vi "MT_generate_signal5.vi"(7 "Direction":bool, 8 "error in (no error)":errorcluster, 9 "# cycles":dbl, 10 "frequency":dbl, 11 "amplitude":dbl) -> (0 "error out":errorcluster, 2 "signals out":dbl[][](array[numeric]), 3 "# samples":dbl)   [LabVIEW 2019]
uses:
  <vilib>/Analysis/NI_AALBase.lvlib
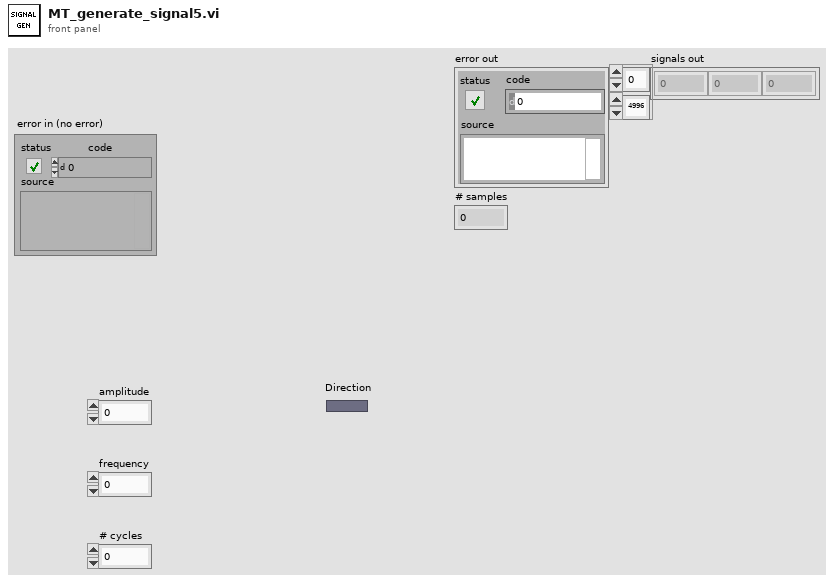
[diagram p1: front panel]
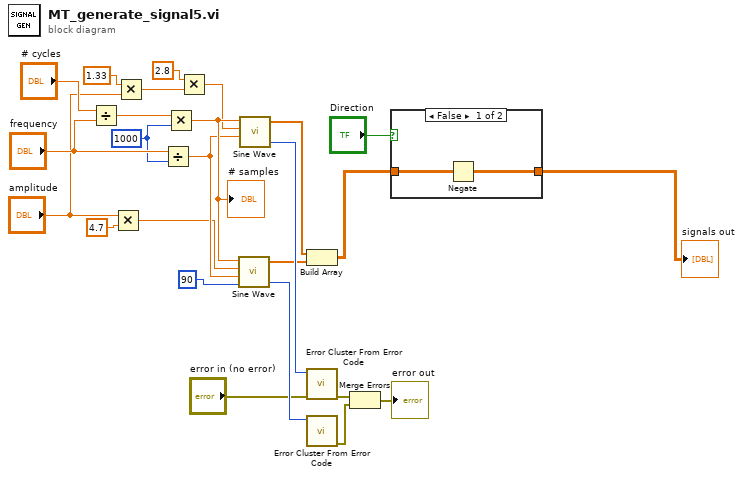
[diagram p0: block diagram]
diagram:
  w22 = 1000
  n1 = Divide(x="# cycles", y="frequency") -> (x/y=w23:dbl)
  n2 = Multiply(x="amplitude", y=4.7) -> (x*y=w18:dbl)
  n3 = Multiply(x=1.33, y="amplitude") -> (x*y=w5:dbl)
  n4 = Divide(x="frequency", y=w22) -> (x/y=w20:dbl)
  n5 = Multiply(x=w23, y=w22) -> (x*y=w21:dbl)
  "# samples" <- w21
  n6 = Multiply(x=2.8, y=w5) -> (x*y=w4:dbl)
  n7 = call <vilib>:"Sine Wave.vi"("samples"=w21, "amplitude"=w18, "frequency"=w20, "phase in"=90) -> ("sine wave"=w7:dbl[], "error"=w16:i32)  [unwired: 1 in, 1 out]
  n8 = call <vilib>:"Sine Wave.vi"("samples"=w21, "amplitude"=w4, "frequency"=w20) -> ("sine wave"=w8:dbl[], "error"=w17:i32)  [unwired: 2 in, 1 out]
  n9 = Build Array(w8, w7) -> (w2:dbl[][])
  n10 = call <vilib>:"Error Cluster From Error Code.vi"("error in (no error)"="error in (no error)", "error code (0)"=w17) -> ("error out"=w14:errorcluster)  [unwired: 7 in]
  n11 = call <vilib>:"Error Cluster From Error Code.vi"("error code (0)"=w16) -> ("error out"=w13:errorcluster)  [unwired: 8 in]
  n12 = Merge Errors(w14, w13) -> (→"error out":errorcluster)
  n13 = case shown="False" "Direction" {
    tunnel: w2 -> [w27 w28]
    tunnel: [w26 w28] -> w1
    frame False {
      n14 = Negate(x=w27) -> (-x=w26:dbl[][])
    }
    frame True {
    }
  }
  "signals out" <- w1
